vi "car3udpmsg_sender.vi"() -> ()   [LabVIEW 2020]
doc: "The UDP protocol differs from TCP in that there is no error-checking with the packets of information that are sent, and thus no guarantee whatsoever that an intended recipient will actually receive a given piece of data.\n\nUDP does offer the ability to \"broadcast\" data across a network--simply specify an IP Address of all ones (255.255.255.255) to attempt to broadcast information network-wide. Keep in mind that routers and other network hardware will generally refuse to forward the broadcast beyond certain points, so the extent of the broadcast will in practice be limited."
panel:
  out "length":i32
  out "message":string
  in  "msg len":u16=35
  in  "target address":string="192.168.232.1:16001"
  in  "from port":u16=16100
  in  "Stop":bool
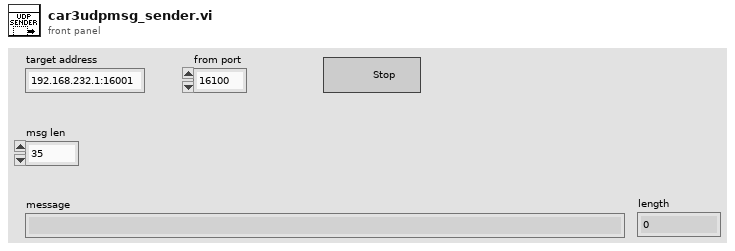
[diagram p1: front panel]
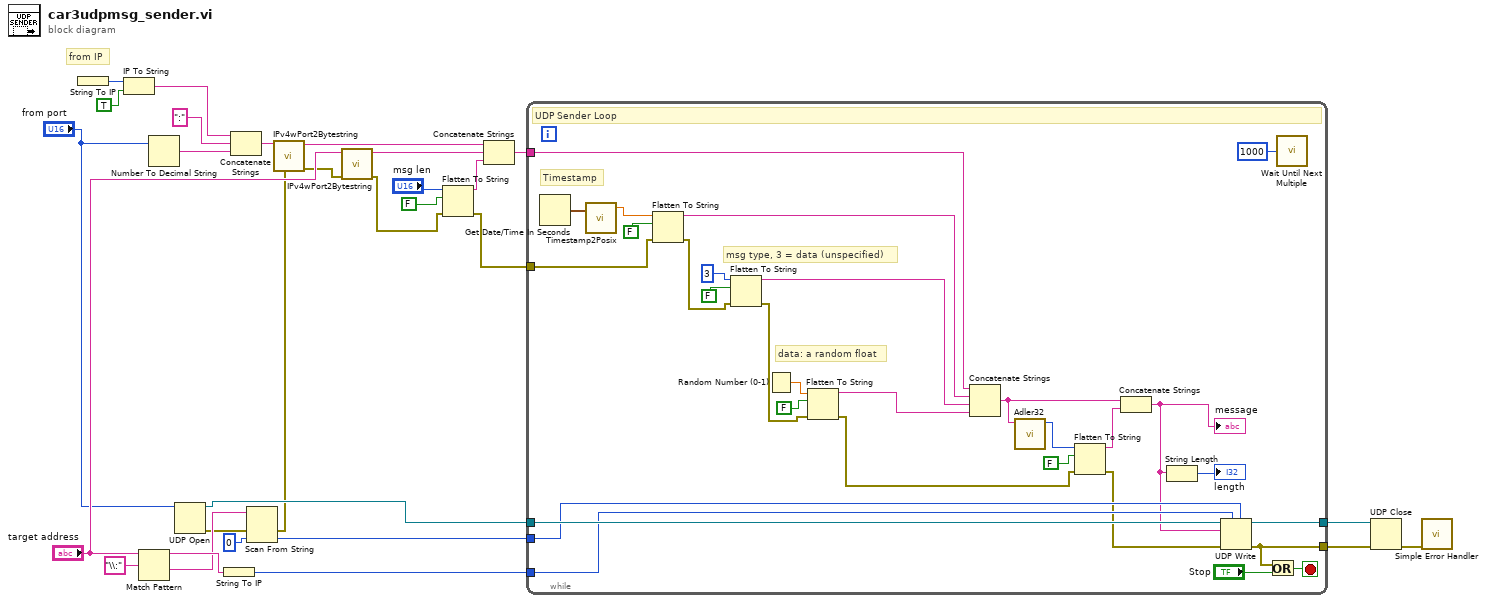
[diagram p0: block diagram]
diagram:
  # "from IP"
  n1 = String To IP() -> (0:w17:u32)  [unwired: 1 in]
  n2 = IP To String(1:TRUE ("dot notation? (F)"), 2:w17) -> (0:w14:string)
  n3 = Match Pattern(string="target address", regular expression="\\:") -> (before substring=w23:string, after substring=w20:string)  [unwired: 1 in, 2 out]
  n4 = Number To Decimal String(number="from port") -> (decimal integer string=w12:string)  [unwired: 1 in]
  n5 = UDP Open(11:"from port") -> (port=w26:refnum<k16>, 0:w19:errorcluster)  [unwired: 4 in, 1 out]
  n6 = String To IP(1:w23) -> (0:w25:u32)
  n7 = Concatenate Strings(w14, ":" ("string"), w12) -> (w11:string)
  n8 = Scan From String(input string=w20, error in=w19, default 1=u16 0 ("from port")) -> (error out=w2:errorcluster, output 1=w21:u16)  [unwired: 2 in, 2 out]
  n9 = call "IPv4wPort2Bytestring.vi"("error in"=w2, "ip address : port"=w11) -> ("error out"=w4:errorcluster, "byte string"=w10:string)  [unwired: 8 in]
  n10 = call "IPv4wPort2Bytestring.vi"("error in"=w4, "ip address : port"="target address") -> ("error out"=w3:errorcluster, "byte string"=w9:string)  [unwired: 8 in]
  n11 = Flatten To String(anything="msg len", prepend array or string size? (T)=FALSE, error in (no error)=w3) -> (data string=w6:string, error out=w1:errorcluster)  [unwired: 1 in, 1 out]
  n12 = Concatenate Strings(w10, w9, w6) -> (w5:string)
  n13 = while {
    tunnel: [w55] -> w28
    tunnel: w26 -> [w59]
    tunnel: [w56] -> w29
    tunnel: w25 -> [w54]
    tunnel: w21 -> [w53]
    tunnel: w5 -> [w49]
    tunnel: w1 -> [w35]
    stop <- w58 stop-if-true
    # "data: a random float"
    # "msg type, 3 = data (unspecified)"
    # "Timestamp"
    # "UDP Sender Loop"
    n14 = Get Date/Time In Seconds() -> (seconds since 1Jan1904=w52:timestamp)
    n15 = call "Timestamp2Posix.vi"("timestamp"=w52) -> ("POSIX"=w50:dbl)  [unwired: 4 in]
    n16 = Flatten To String(anything=w50, prepend array or string size? (T)=FALSE, error in (no error)=w35) -> (data string=w48:string, error out=w34:errorcluster)  [unwired: 1 in, 1 out]
    n17 = Flatten To String(anything=u8 3, prepend array or string size? (T)=FALSE, error in (no error)=w34) -> (data string=w44:string, error out=w33:errorcluster)  [unwired: 1 in, 1 out]
    n18 = Random Number (0-1)() -> (number: 0 to 1=w36:dbl)
    n19 = Flatten To String(anything=w36, prepend array or string size? (T)=FALSE, error in (no error)=w33) -> (data string=w43:string, error out=w32:errorcluster)  [unwired: 1 in, 1 out]
    n20 = Concatenate Strings(w49, w48, w44, w43) -> (w40:string)
    n21 = call "Adler32.vi"("input_string"=w40) -> ("Adler32"=w39:u32)  [unwired: 10 in]
    n22 = Flatten To String(anything=w39, prepend array or string size? (T)=FALSE, error in (no error)=w32) -> (data string=w41:string, error out=w31:errorcluster)  [unwired: 1 in, 1 out]
    n23 = Concatenate Strings(w40, w41) -> (w38:string)
    "message" <- w38
    n24 = String Length(string=w38) -> (length=→"length":i32)
    n25 = UDP Write(address=w54, port or service name=w53, connection ID=w59, data in=w38, 8:w31) -> (error out=w55:errorcluster, 3:w56:refnum<k16>)  [unwired: 1 in]
    n26 = Or(x=w55, y="Stop") -> (x .or. y?=w58:bool)
    n27 = call "Wait Until Next Multiple"("Count(mSec)"=u32 1000 ("millisecond multiple")) -> ()  [unwired: 1 out]
  }
  n28 = UDP Close(connection ID=w29, 8:w28) -> (error out=w27:errorcluster)  [unwired: 1 out]
  n29 = call <vilib>:"Simple Error Handler.vi"("error in (no error)"=w27) -> ()  [unwired: 4 in, 5 out]
